vi "ImagingAndControl.vi"() -> ()   [LabVIEW 2015]
uses:
  <userlib>/atmcd64d.llb/Error Code Enum typedef.ctl
  <userlib>/atmcd64d.llb/HSSpeed_type typedef.ctl
  <vilib>/Analysis/baseanly.llb/Mean (DBL).vi
  AcquisitionGlobals.vi
  NIDAQControls/StateGlobals.vi
  NIDAQControls/NIDAQGlobals.vi
  LiveImage_Global.vi
  StartupVI_Globals.vi
  <userlib>/AB_ALC_REV64/AB_ALC_REV64.lvlib
  <vilib>/Analysis/NI_AALBase.lvlib
panel:
  out "gain":u32
  in  "Set EM Gain":u16(slide)=2995 min=3 max=300 scale=0.8..300.0
  in  "Live Volume":bool
  in  "max ypixels":i32=512
  in  "max xpixels":i32=512
  out "Saving?":bool
  out "Exposure Out":dbl=10.0
  out "start time":dbl format="%_19f"
  out "status":T1=enum."DRV_TEMPERATURE_STABILIZED"
  out "temperature":i32=-71
  in  "Acq Speed":u16(ring) items=["17", "10", "5", "1"]
  in  "Filter Position":i8=5
  out "Acquiring?":bool
  in  "ypixels":i32=512
  in  "xpixels":i32=512
  out "error out":errorcluster={"status"=FALSE, "code"=5002, "source"="ImagingAndControl.vi->GetAcquisitionTimings.vi"}
  in  "Tab Control":enum32{"Piezo Control", "Laser Control"}(tab)
  in  "Abort!":bool
  out "Recording time":dbl=16.0 format="%<%H:%M:%S%2u>t"
  out "Num Slices":u16=16
  in  "Waveform Type":enum16{"Triangle", "Sawtooth"}(ring)=enum."Sawtooth"
  in  "Center Piezo":bool
  out "Recording Progress":u8(slide) scale=0.0..100.0
  in  "Begin Acquisition":bool
  in  "File to Save":path=path "E:/maggot images/Jacob/Test/test_run143"
  in  "Acquisition Time (sec)":dbl=120.0
  in  "Volume On/Off":bool=TRUE
  out "Improper \nRange!":bool
  in  "Z Step Size (um)":dbl=0.8
  out "Current Z Position (um)":dbl=46.25
  in  "Max (um)":dbl=52.0
  in  "Min (um)":dbl=40.5
  in  "Set Min Piezo":bool
  in  "Set Max Piezo":bool
  out "Piezo Position":dbl(slide)=46.25 scale=0.0..100.0
  in  "Piezo Dwell":u16=1
  in  "Piezo Offset":dbl=-0.01
  out "Data Write Progress":u8(slide) scale=0.0..100.0
  in  "Trigger Mode":enum16{"Normal", "One Red Frame Per Volume"}(ring)=enum."One Red Frame Per Volume"
  in  "AOTF3 - 561 nm":dbl(slide)=21.02803738317757 scale=0.0..100.0
  in  "AOTF2 - 488 nm":dbl(slide)=20.560747663551403 scale=0.0..100.0
  in  "AOTF1 - 440 nm":dbl(slide) scale=0.0..100.0
  in  "Initialize Things?":bool
  out "Laser Mode":string="Confocal Green"
  in  "Live":bool
  in  "Exposure Time":T2(ring)
  in  "Triggered":bool
  in  "Confocal Red":bool
  in  "Confocal Green":bool=TRUE
  in  "Confocal Blue":bool
  out "LaserID":i32=2
  in  "stop":bool
  # ".h5"
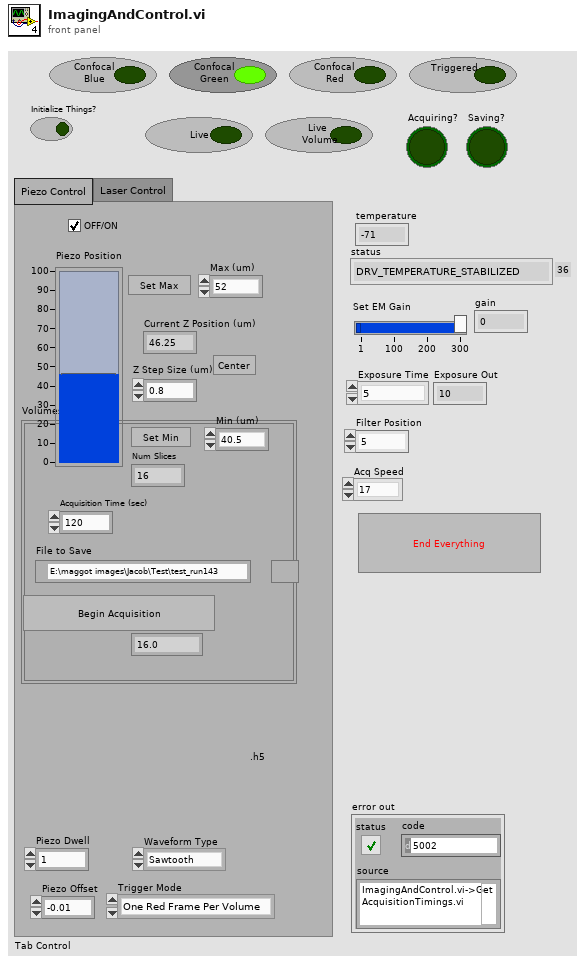
[diagram p1: front panel]
types:
  T1 = typedef "Error Code Enum typedef.ctl" = enum32{"N/A (0)", "DRV_ERROR_CODES", "DRV_SUCCESS", "DRV_VXDNOTINSTALLED", "DRV_ERROR_SCAN", "DRV_ERROR_CHECK_SUM", "DRV_ERROR_FILELOAD", "DRV_UNKNOWN_FUNC", "DRV_ERROR_VXD_INIT", "DRV_ERROR_ADDRESS", "DRV_ERROR_PAGELOCK", "DRV_ERROR_PAGEUNLOCK", "DRV_ERROR_BOARDTEST", "DRV_ERROR_ACK", "DRV_ERROR_UP_FIFO", "DRV_ERROR_PATTERN", "N/A (16)", "DRV_ACQUISITION_ERRORS", "DRV_ACQ_BUFFER", "DRV_ACQ_DOWNFIFO_FULL", "DRV_PROC_UNKONWN_INSTRUCTION", "DRV_ILLEGAL_OP_CODE", "DRV_KINETIC_TIME_NOT_MET", "DRV_ACCUM_TIME_NOT_MET", "DRV_NO_NEW_DATA", "N/A (25)", "DRV_SPOOLERROR", "N/A (27)", "N/A (28)", "N/A (29)", "N/A (30)", "N/A (31)", "N/A (32)", "DRV_TEMPERATURE_CODES", "DRV_TEMPERATURE_OFF", "DRV_TEMPERATURE_NOT_STABILIZED", "DRV_TEMPERATURE_STABILIZED", "DRV_TEMPERATURE_NOT_REACHED", "DRV_TEMPERATURE_OUT_RANGE", "DRV_TEMPERATURE_NOT_SUPPORTED", "DRV_TEMPERATURE_DRIFT", "N/A (41)", "N/A (42)", "N/A (43)", "N/A (44)", "N/A (45)", "N/A (46)", "N/A (47)", "N/A (48)", "DRV_GENERAL_ERRORS", "DRV_INVALID_AUX", "DRV_COF_NOTLOADED", "DRV_FPGAPROG", "DRV_FLEXERROR", "DRV_GPIBERROR", "N/A (55)", "N/A (56)", "N/A (57)", "N/A (58)", "N/A (59)", "N/A (60)", "N/A (61)", "N/A (62)", "N/A (63)", "DRV_DATATYPE", "DRV_DRIVER_ERRORS", "DRV_P1INVALID", "DRV_P2INVALID", "DRV_P3INVALID", "DRV_P4INVALID", "DRV_INIERROR", "DRV_COFERROR", "DRV_ACQUIRING", "DRV_IDLE", "DRV_TEMPCYCLE", "DRV_NOT_INITIALIZED", "DRV_P5INVALID", "DRV_P6INVALID", "DRV_INVALID_MODE", "DRV_INVALID_FILTER", "DRV_I2CERRORS", "DRV_I2CDEVNOTFOUND", "DRV_I2CTIMEOUT", "DRV_P7INVALID", "N/A (84)", "N/A (85)", "N/A (86)", "N/A (87)", "N/A (88)", "N/A (89)", "DRV_IOCERROR", "DRV_VRMVERSIONERROR"}
  T2 = enum16{"5", "10", "15", "20", "25", "30", "35", "40", "50", "60", "70", "100", "500"}
  T3 = cluster{"Start or New Parameters?":bool, "Laser Mode":string, "Piezo Mode":string, "Begin Or End Acquisition":string, "Acquisition Time":dbl}
  T4 = enum8{"Enabled", "Disabled", "Disabled and Grayed Out"}
  T5 = enum32{"Invalid", "Standard", "Closed", "Hidden", "Minimized", "Maximized"}
  T6 = typedef "HSSpeed_type typedef.ctl" = enum16{"EM Amp", "Conventional Amp"}
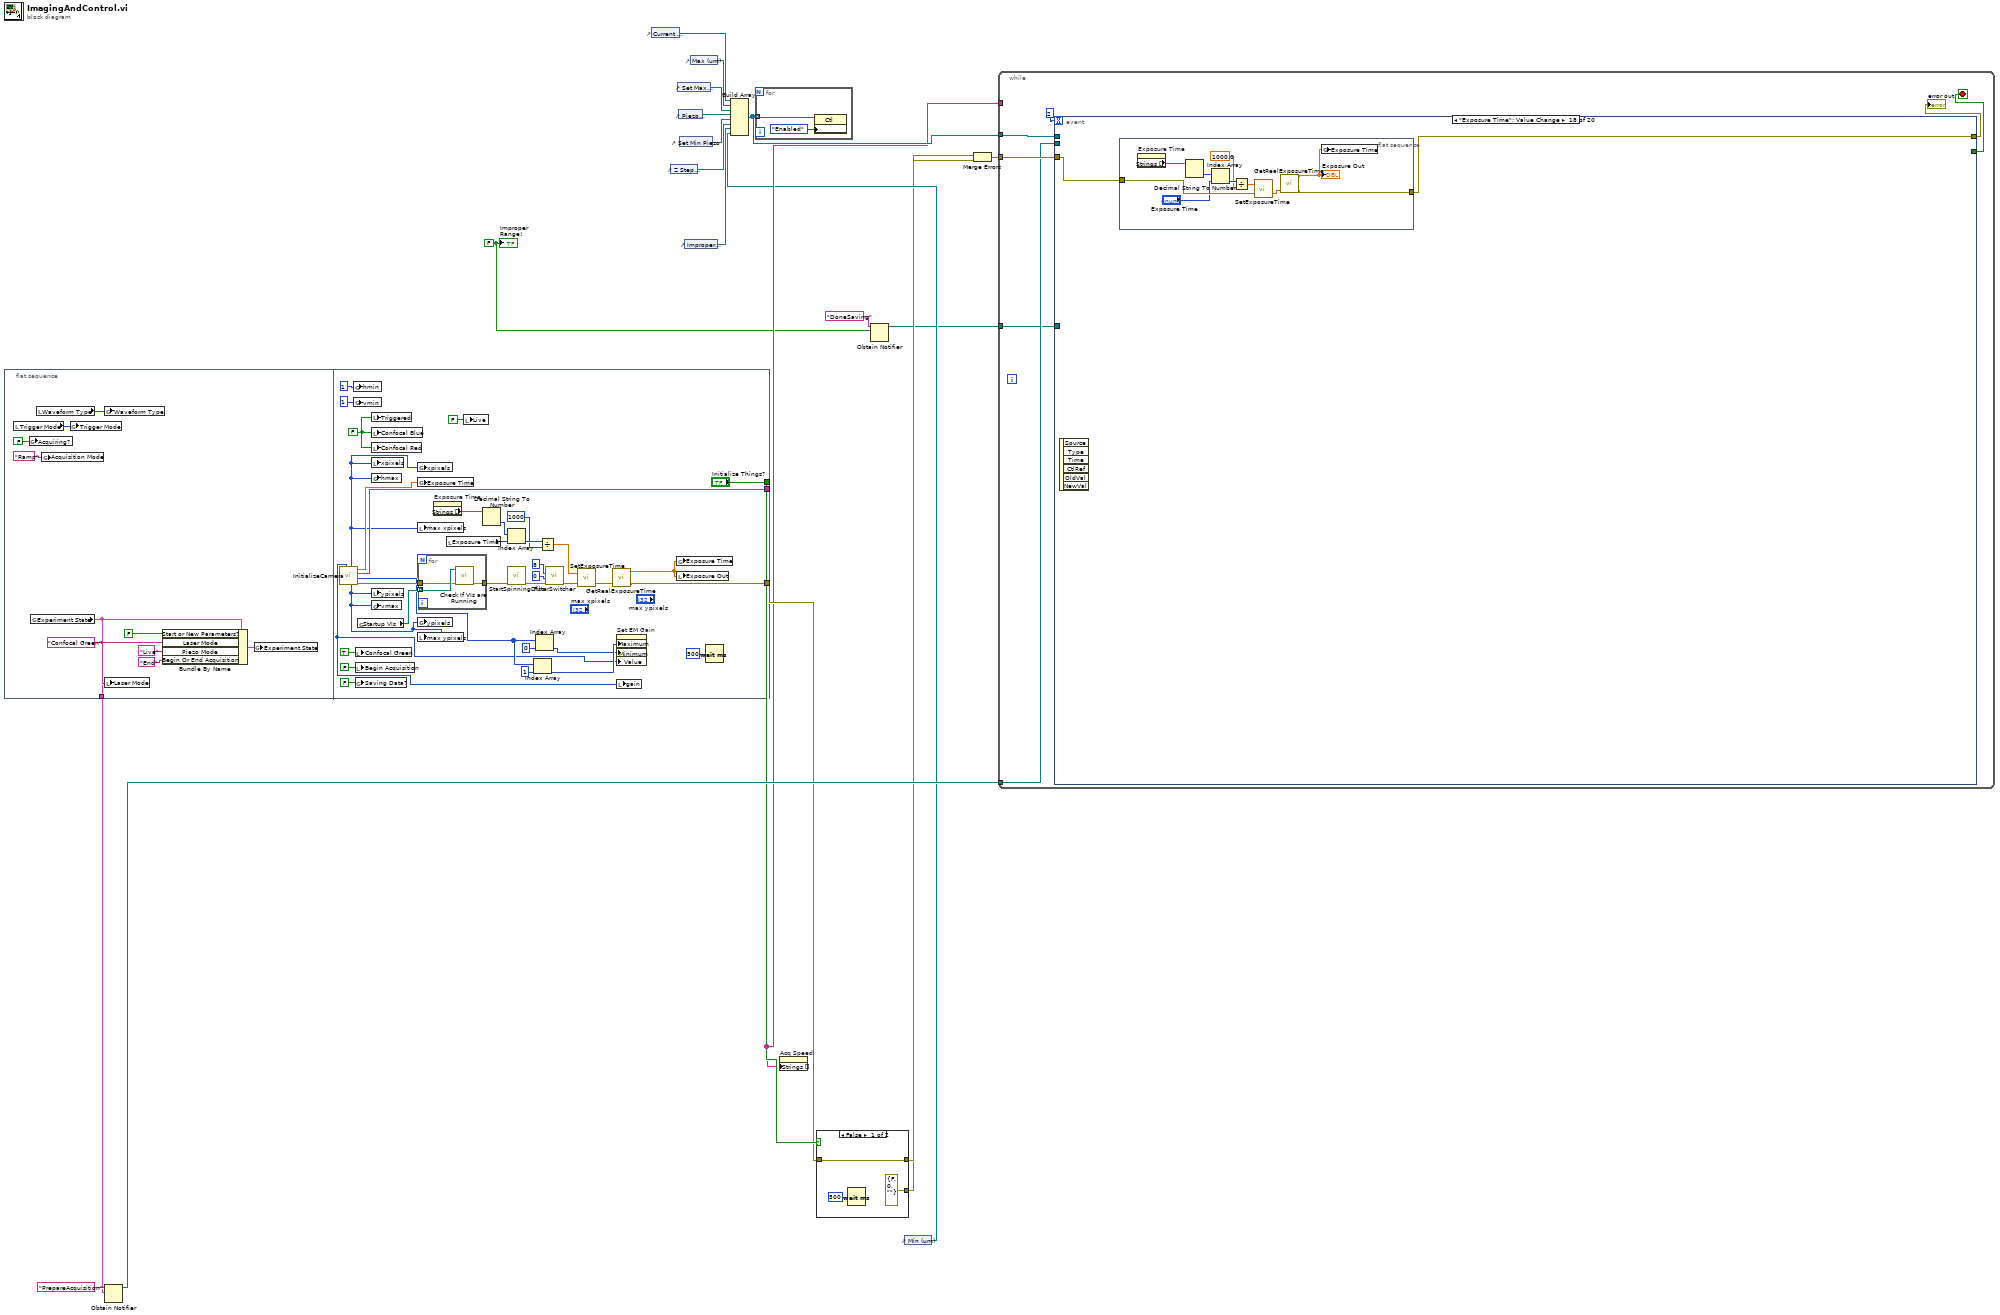
[diagram p0: block diagram]
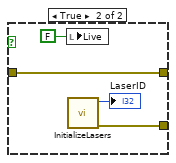
[diagram p2: hidden frame]
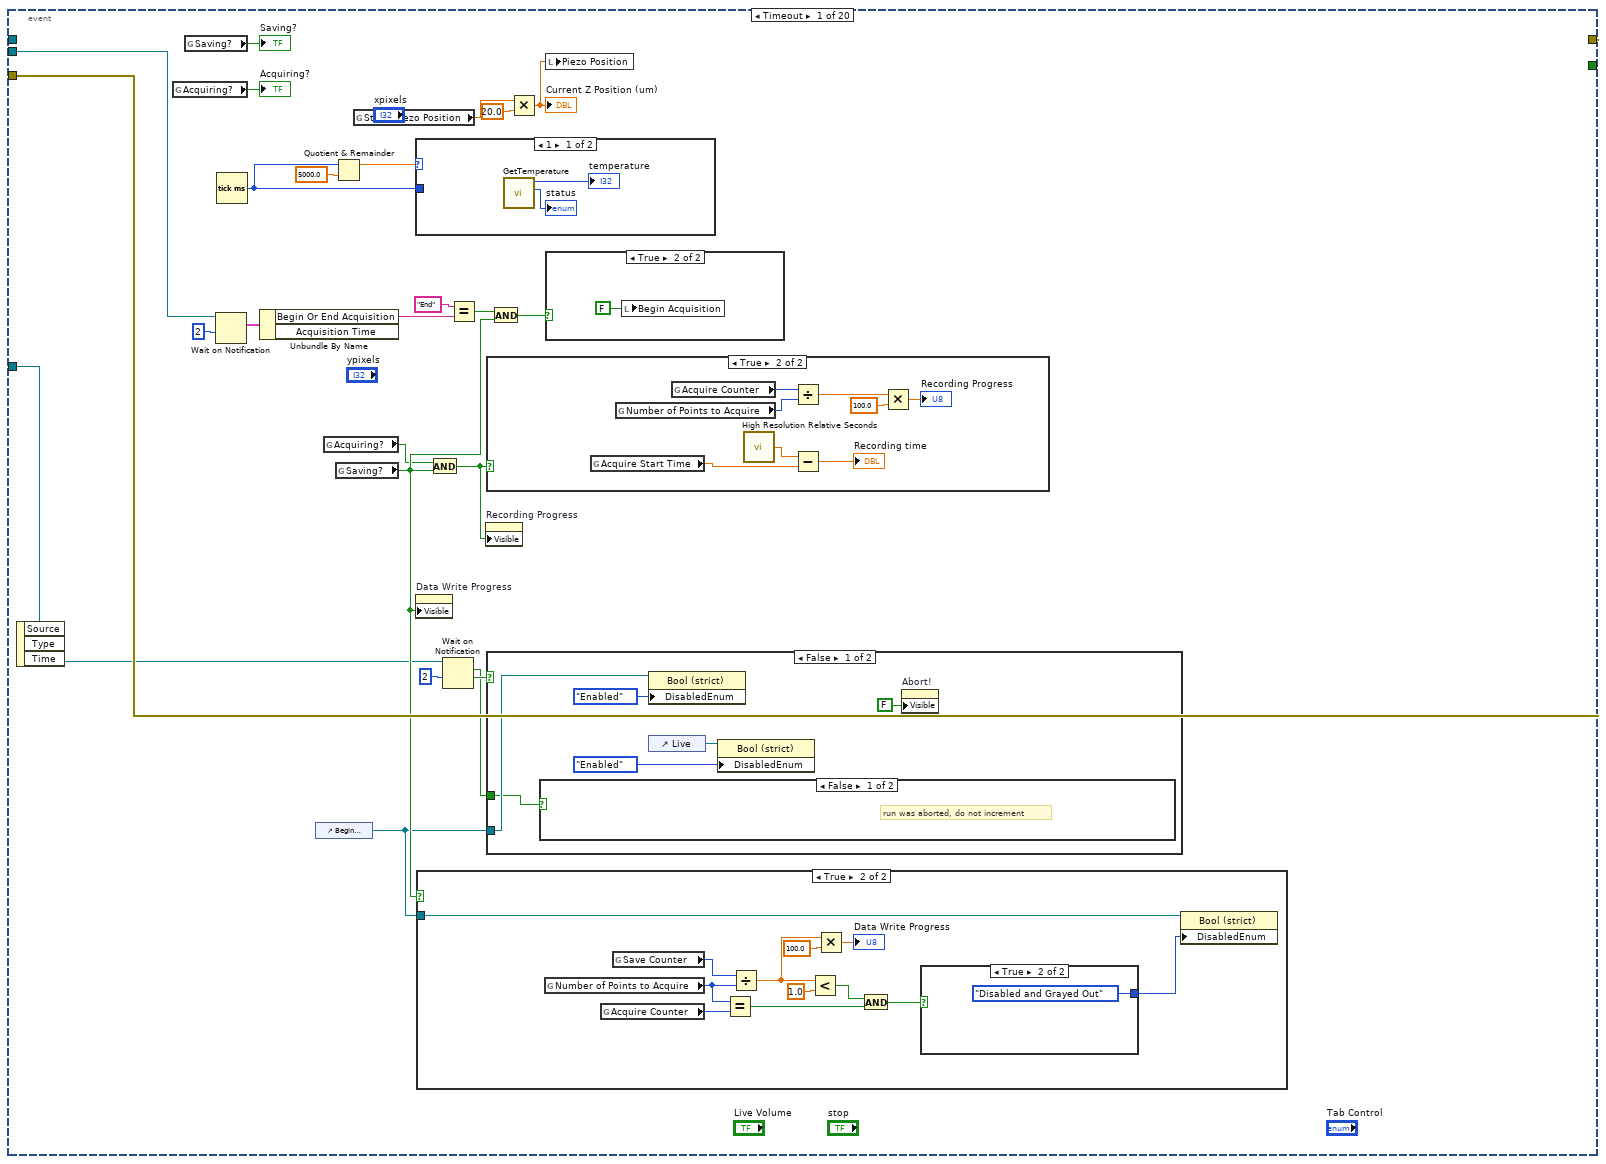
[diagram p3: hidden frame]
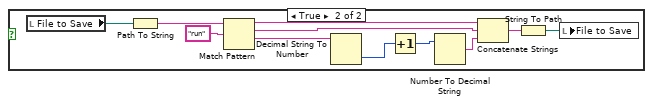
[diagram p4: hidden frame]
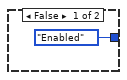
[diagram p8: hidden frame]
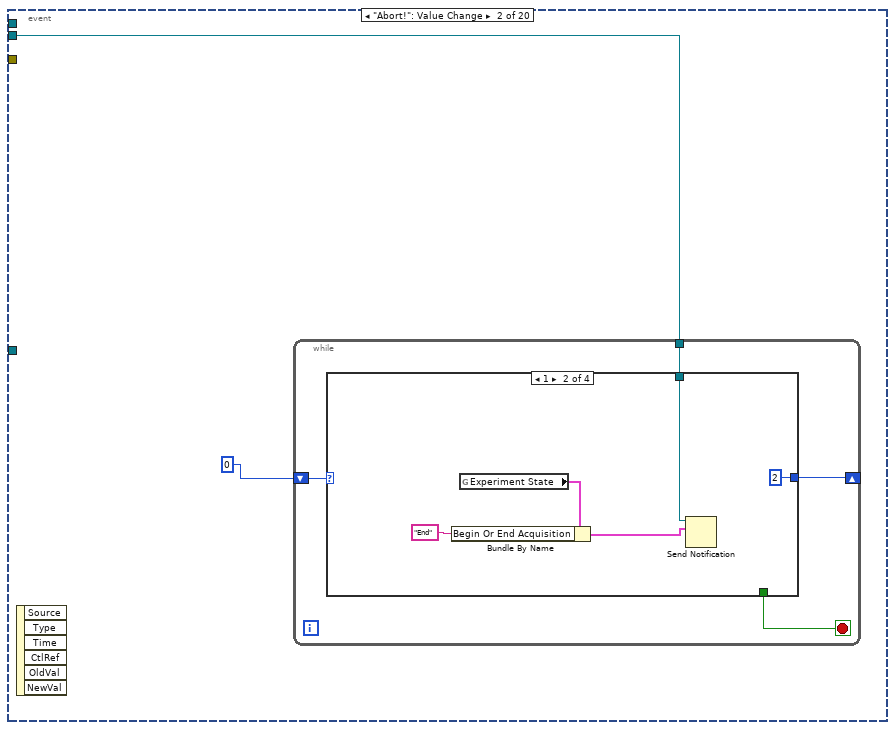
[diagram p11: hidden frame]
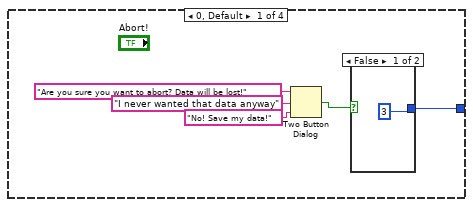
[diagram p12: hidden frame]
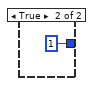
[diagram p13: hidden frame]
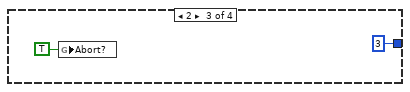
[diagram p14: hidden frame]
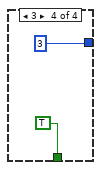
[diagram p15: hidden frame]
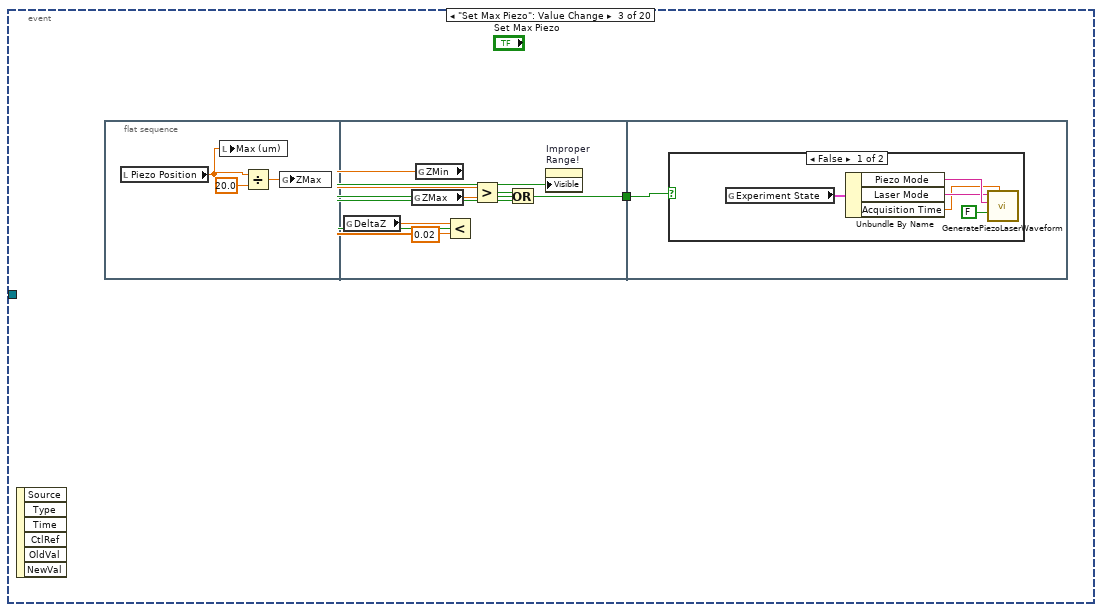
[diagram p16: hidden frame]
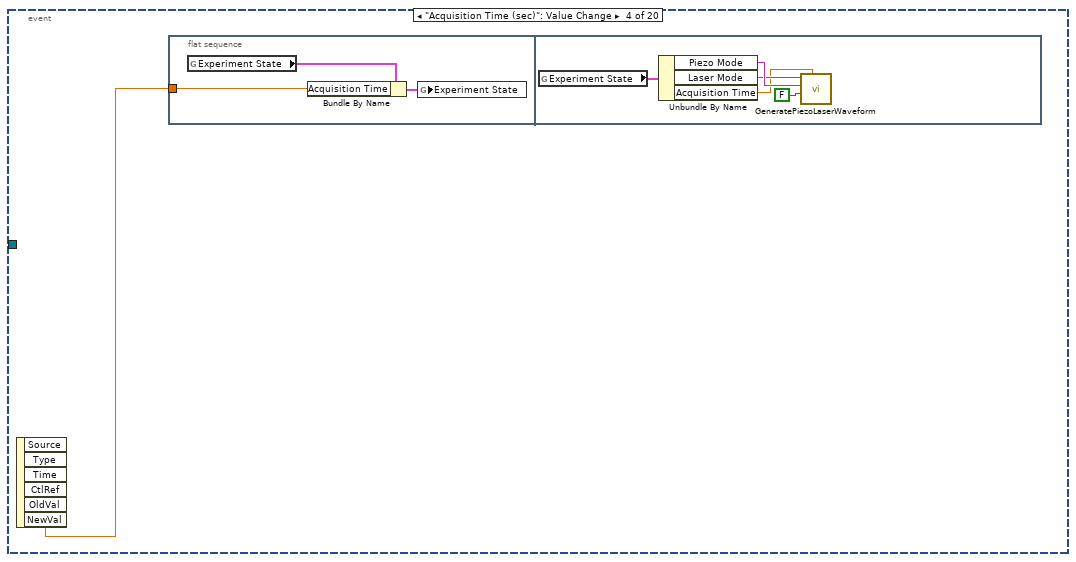
[diagram p18: hidden frame]
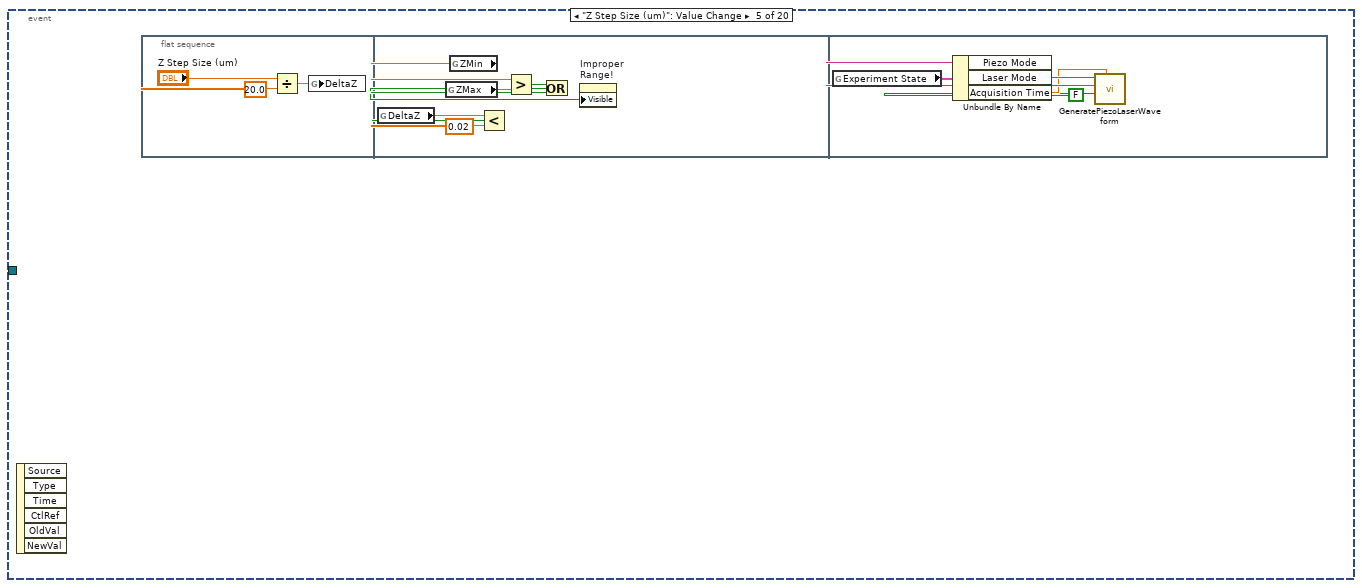
[diagram p19: hidden frame]
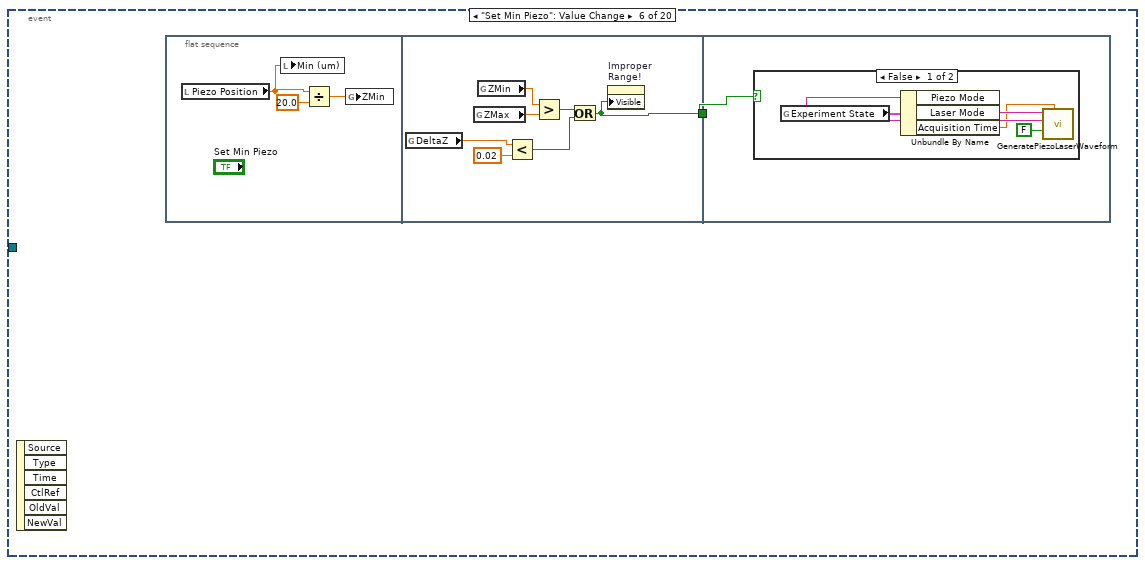
[diagram p20: hidden frame]
diagram:
  w2 = FALSE ("Improper \nRange!")
  n1 = flat-sequence {
    tunnel: [w24] -> w8
    tunnel: ["Initialize Things?"] -> w19
    tunnel: [w33] -> w10
    tunnel: [w56] -> w9
    frame #0 {
      w26 = "Confocal Green" ("Laser Mode")
      n2 = local read "Trigger Mode"() -> (w23:enum16{"Normal", "One Red Frame Per Volume"})
      n3 = global write "AcquisitionGlobals.vi" "Acquiring?"(FALSE ("Acquiring?")) -> ()
      n4 = global read "StateGlobals.vi" "Experiment State"() -> (w24:T3)
      n5 = local read "Waveform Type"() -> (w22:enum16{"Triangle", "Sawtooth"})
      n6 = global write "AcquisitionGlobals.vi" "Acquisition Mode"("Ramp" ("Acquisition Mode")) -> ()
      n7 = global write "NIDAQGlobals.vi" "Trigger Mode"(w23) -> ()
      n8 = global write "NIDAQGlobals.vi" "Waveform Type"(w22) -> ()
      n9 = local write "Laser Mode"(w26) -> ()
      n10 = Bundle By Name(cluster=w24, "Start or New Parameters?"=FALSE, "Laser Mode"=w26, "Piezo Mode"="Live", "Begin Or End Acquisition"="End") -> (w28:T3)
      n11 = global write "StateGlobals.vi" "Experiment State"(w28) -> ()
    }
    frame #1 {
      w61 = FALSE ("Confocal Blue")
      n12 = call "InitializeCamera.vi"() -> ("error out"=w64:errorcluster, "EM Gain Range"=w38:i32[], "EM Speeds"=w56:string[], "exposure time"=w60:sgl, "ypixels"=w52:i32, "xpixels"=w54:i32, "EM Gain"=w35:u32)  [unwired: 5 in]
      n13 = global write "LiveImage_Global.vi" "hmin"(1 ("hmin")) -> ()
      n14 = global write "LiveImage_Global.vi" "vmin"(1 ("vmin")) -> ()
      n15 = local write "Confocal Green"(TRUE ("Confocal Green")) -> ()
      n16 = local write "Begin Acquisition"(FALSE ("Begin Acquisition")) -> ()
      n17 = global write "AcquisitionGlobals.vi" "Saving Data?"(FALSE ("Saving Data?")) -> ()
      n18 = global read "StartupVI_Globals.vi" "Startup VIs"() -> (w65:path[])
      n19 = local write "Triggered"(w61) -> ()
      n20 = local write "Confocal Blue"(w61) -> ()
      n21 = local write "Confocal Red"(w61) -> ()
      n22 = local write "xpixels"(w54) -> ()
      n23 = global write "LiveImage_Global.vi" "hmax"(w54) -> ()
      n24 = local write "ypixels"(w52) -> ()
      n25 = global write "LiveImage_Global.vi" "vmax"(w52) -> ()
      n26 = global write "LiveImage_Global.vi" "xpixels"(w54) -> ()
      n27 = global write "LiveImage_Global.vi" "Exposure Time"(w60) -> ()
      n28 = local write "max xpixels"(w54) -> ()
      n29 = for {
        tunnel: w65 -> [w69] mode=indexing
        tunnel: w64 -> [w68]
        tunnel: [w67] -> w62
        n30 = call "Check If VIs are Running.vi"("error in (no error)"=w68, "Path"=w69) -> ("error out"=w67:errorcluster)  [unwired: 9 in]
      }
      n31 = global write "LiveImage_Global.vi" "ypixels"(w52) -> ()
      n32 = local write "max ypixels"(w52) -> ()
      n33 = property on="Exposure Time" class="Enum (strict)"() -> ("Strings []"=w47:string[])  [unwired: 2 in, 2 out]
      n34 = local read "Exposure Time"() -> (w46:T2)
      n35 = local write "Live"(FALSE ("Live")) -> ()
      n36 = Decimal String To Number(string=w47) -> (number=w49:i32[])  [unwired: 2 in, 1 out]
      n37 = Index Array(array=w49, index=w46) -> (element=w48:i32)
      n38 = call "StartSpinningDisc.vi"("error in (no error)"=w62) -> ("error out"=w59:errorcluster)  [unwired: 10 in]
      n39 = Index Array(array=w38, index=1) -> (element=w37:i32)
      n40 = Index Array(array=w38, index=0) -> (element=w36:i32)
      n41 = Divide(x=w48, y=1000) -> (x/y=w45:dbl)
      n42 = call "FilterSwitcher.vi"("error in (no error)"=w59, "Filter Change Speed"=0, "Filter Position"=8) -> ("error out"=w50:errorcluster)  [unwired: 8 in]
      n43 = call <userlib>:"SetExposureTime.vi"("error in (no error)"=w50, "time"=w45) -> ("error out"=w34:errorcluster)  [unwired: 1 out]
      n44 = call "GetRealExposureTime.vi"("error in (no error)"=w34) -> ("error out"=w33:errorcluster, "Actual Exposure Time (ms)"=w32:dbl)  [unwired: 9 in]
      n45 = property on="Set EM Gain" class="Slide (strict)"("Maximum"=w37, "Minimum"=w36, "Value"=w35) -> ()  [unwired: 2 in, 2 out]
      n46 = local write "gain"(w35) -> ()
      n47 = global write "LiveImage_Global.vi" "Exposure Time"(w32) -> ()
      n48 = local write "Exposure Out"(w32) -> ()
      n49 = Wait (ms)(milliseconds to wait=u32 500) -> ()  [unwired: 1 out]
    }
  }
  n50 = Obtain Notifier(name (unnamed)="PrepareAcquisition", notification data type=w8) -> (notifier out=w20:refnum<notifier>)  [unwired: 2 in, 2 out]
  n51 = control-ref of="Current Z Position (um)"() -> (w18:refnum<vi>)
  n52 = control-ref of="Z Step Size (um)"() -> (w13:refnum<vi>)
  n53 = control-ref of="Set Max Piezo"() -> (w16:refnum<vi>)
  n54 = control-ref of="Piezo Position"() -> (w15:refnum<vi>)
  n55 = control-ref of="Set Min Piezo"() -> (w14:refnum<vi>)
  n56 = control-ref of="Improper \nRange!"() -> (w12:refnum<vi>)
  n57 = control-ref of="Max (um)"() -> (w17:refnum<vi>)
  n58 = property on="Acq Speed" class="Ring (strict)"("Strings []"=w9) -> ()  [unwired: 2 in, 2 out]
  n59 = case shown="False" w19 {
    tunnel: [w71 w76] -> w6
    tunnel: [errorcluster {"status"=FALSE, "code"=0, "source"=""} ("error out") w75] -> w5
    tunnel: w10 -> [w71 w76]
    frame False {
      n60 = Wait (ms)(milliseconds to wait=u32 500) -> ()  [unwired: 1 out]
    }
    frame True {
      n61 = local write "Live"(FALSE ("Live")) -> ()
      n62 = call "InitializeLasers.vi"() -> ("error out"=w75:errorcluster, "hALC_REV out"=→"LaserID":i32)  [unwired: 10 in]
    }
  }
  n63 = Obtain Notifier(name (unnamed)="DoneSaving", notification data type=w2) -> (notifier out=w1:refnum<notifier>)  [unwired: 2 in, 2 out]
  n64 = control-ref of="Min (um)"() -> (w7:refnum<vi>)
  n65 = Build Array(w18, w17, w16, w15, w14, w13, w12, w7) -> (w11:refnum<vi>[])
  n66 = for {
    tunnel: w11 -> [w78] mode=indexing
    n67 = property class="Ctl"(reference=w78, "DisabledEnum"=T4."Enabled" ("Disabled")) -> ()  [unwired: 1 in, 2 out]
  }
  n68 = Merge Errors(w5, w6) -> (w4:errorcluster)
  n69 = while {
    tunnel: w4 -> [w85]
    tunnel: w20 -> [w84]
    tunnel: w11 -> [w82]
    tunnel: w9 -> [_]
    tunnel: w1 -> [w79]
    stop <- w81 stop-if-true
    n70 = event shown="[17] \"Exposure Time\": Value Change" {
      selector: _ -> [_ _ _ _ _ _ _ _ _ _ _ _ _ _ _ _ _ _ _ _]
      dyn-events: _ -> [_ _ _ _ _ _ _ _ _ _ _ _ _ _ _ _ _ _ _ _]
      timeout: 2 -> [_ _ _ _ _ _ _ _ _ _ _ _ _ _ _ _ _ _ _ _]
      tunnel: w85 -> [w94 _ _ _ _ _ w233 w263 w282 _ w308 w323 w326 w375 _ w442 _ w468 w483 _]
      tunnel: [w94 _ _ _ _ _ w232 w262 w281 _ w306 _ w324 w371 _ w441 _ w467 w483 _] -> w83
      tunnel: [_ _ _ _ _ _ _ _ _ _ w303 _ _ _ _ _ _ _ _ _] -> w81
      tunnel: w84 -> [w102 w152 _ _ _ _ w234 w264 w283 _ _ _ w325 w377 _ _ w449 _ w481 w503]
      tunnel: w82 -> [_ _ _ _ _ _ _ _ _ w296 _ _ _ _ _ _ _ _ _ _]
      tunnel: w79 -> [w90 _ _ _ _ _ _ _ _ _ _ _ _ _ _ _ _ _ _ _]
      event Timeout {
        n71 = event-data() -> ()  [unwired: 1 in, 3 out]
        n72 = global read "AcquisitionGlobals.vi" "Acquiring?"() -> (→"Acquiring?":bool)
        n73 = global read "AcquisitionGlobals.vi" "Saving?"() -> (→"Saving?":bool)
        n74 = Wait on Notification(notifier=w102, timeout in ms (-1)=2) -> (notification=w101:T3)  [unwired: 2 in, 3 out]
        n75 = Tick Count (ms)() -> (millisecond timer value=w105:u32)
        n76 = Unbundle By Name(w101) -> ("Begin Or End Acquisition"=w99:string)  [unwired: 1 out]
        n77 = control-ref of="Begin Acquisition"() -> (w87:refnum<vi>)
        n78 = global read "AcquisitionGlobals.vi" "Acquiring?"() -> (w92:bool)
        n79 = Quotient & Remainder(x=w105, y=5000.0) -> (x-y*floor(x/y)=w104:dbl)  [unwired: 1 out]
        n80 = global read "AcquisitionGlobals.vi" "Saving?"() -> (w93:bool)
        n81 = global read "NIDAQGlobals.vi" "Static Piezo Position"() -> (w109:dbl)
        n82 = case shown="1" w104 {
          tunnel: w105 -> [_ _]
          frame 1 {
            n83 = call <userlib>:"GetTemperature.vi"() -> ("status"=→"status":T1, "temperature"=→"temperature":i32)  [unwired: 4 in, 2 out]
          }
          frame 0, Default {
          }
        }
        n84 = property on="Data Write Progress" class="Slide (strict)"("Visible"=w93) -> ()  [unwired: 2 in, 2 out]
        n85 = case shown="True" w93 {
          tunnel: w87 -> [_ w135]
          frame False {
          }
          frame True {
            n86 = global read "StateGlobals.vi" "Number of Points to Acquire"() -> (w137:i32)
            n87 = global read "StateGlobals.vi" "Acquire Counter"() -> (w138:i32)
            n88 = global read "StateGlobals.vi" "Save Counter"() -> (w144:i32)
            n89 = Equal?(x=w137, y=w138) -> (x = y?=w140:bool)
            n90 = Divide(x=w144, y=w137) -> (x/y=w143:dbl)
            n91 = Less?(x=w143, y=1.0) -> (x < y?=w141:bool)
            n92 = Multiply(x=w143, y=100.0) -> (x*y=→"Data Write Progress":dbl)
            n93 = And(x=w141, y=w140) -> (x .and. y?=w139:bool)
            n94 = case shown="True" w139 {
              tunnel: [T4."Enabled" ("Disabled") T4."Disabled and Grayed Out" ("Disabled")] -> w136
              frame False {
              }
              frame True {
              }
            }
            n95 = property class="Bool (strict)"(reference=w135, "DisabledEnum"=w136) -> ()  [unwired: 1 in, 2 out]
          }
        }
        n96 = And(x=w92, y=w93) -> (x .and. y?=w91:bool)
        n97 = Wait on Notification(notifier=w90, timeout in ms (-1)=2) -> (notification=w86:bool, timed out?=w88:bool)  [unwired: 2 in, 2 out]
        n98 = Equal?(x="End", y=w99) -> (x = y?=w98:bool)
        n99 = property on="Recording Progress" class="Slide (strict)"("Visible"=w91) -> ()  [unwired: 2 in, 2 out]
        n100 = case shown="True" w91 {
          frame False {
          }
          frame True {
            n101 = global read "StateGlobals.vi" "Acquire Start Time"() -> (w129:dbl)
            n102 = global read "StateGlobals.vi" "Number of Points to Acquire"() -> (w128:i32)
            n103 = global read "StateGlobals.vi" "Acquire Counter"() -> (w127:i32)
            n104 = call <vilib>:"High Resolution Relative Seconds.vi"() -> ("relative seconds"=w134:dbl)
            n105 = Divide(x=w127, y=w128) -> (x/y=w130:dbl)
            n106 = Subtract(x=w134, y=w129) -> (x-y=→"Recording time":dbl)
            n107 = Multiply(x=w130, y=100.0) -> (x*y=→"Recording Progress":dbl)
          }
        }
        n108 = case shown="False" w88 {
          tunnel: w87 -> [w112 _]
          tunnel: w86 -> [w110 _]
          frame False {
            n109 = case shown="False" w110 {
              frame False {
                # "run was aborted, do not increment"
              }
              frame True {
                n110 = local read "File to Save"() -> (w116:path)
                n111 = Path To String(path=w116) -> (string=w118:string)
                n112 = Match Pattern(string=w118, regular expression="run") -> (before substring=w122:string, match substring=w123:string, after substring=w119:string)  [unwired: 1 in, 1 out]
                n113 = Decimal String To Number(string=w119) -> (number=w120:i32)  [unwired: 2 in, 1 out]
                n114 = Increment(x=w120) -> (x+1=w121:i32)
                n115 = Number To Decimal String(number=w121) -> (decimal integer string=w124:string)  [unwired: 1 in]
                n116 = Concatenate Strings(w122, w123, w124) -> (w125:string)
                n117 = String To Path(string=w125) -> (path=w126:path)
                n118 = local write "File to Save"(w126) -> ()
              }
            }
            n119 = property class="Bool (strict)"(reference=w112, "DisabledEnum"=T4."Enabled" ("Disabled")) -> ()  [unwired: 1 in, 2 out]
            n120 = control-ref of="Live"() -> (w113:refnum<vi>)
            n121 = property class="Bool (strict)"(reference=w113, "DisabledEnum"=T4."Enabled" ("Disabled")) -> ()  [unwired: 1 in, 2 out]
            n122 = property on="Abort!" class="Bool (strict)"("Visible"=FALSE) -> ()  [unwired: 2 in, 2 out]
          }
          frame True {
          }
        }
        n123 = And(x=w98, y=w93) -> (x .and. y?=w95:bool)
        n124 = Multiply(x=w109, y=20.0) -> (x*y=w107:dbl)
        "Current Z Position (um)" <- w107
        n125 = local write "Piezo Position"(w107) -> ()
        n126 = case shown="True" w95 {
          frame False {
          }
          frame True {
            n127 = local write "Begin Acquisition"(FALSE ("Begin Acquisition")) -> ()
          }
        }
      }
      event "Abort!": Value Change {
        n128 = event-data() -> ()  [unwired: 1 in, 6 out]
        n129 = while {
          shift-right: [w156] -> _
          shift-left: 0 -> [w157]
          tunnel: w152 -> [w154]
          stop <- w155 stop-if-true
          n130 = case shown="1" w157 {
            tunnel: [w158 2 3 3] -> w156
            tunnel: [_ _ _ TRUE] -> w155
            tunnel: w154 -> [_ w166 _ _]
            frame 0, Default {
              n131 = Two Button Dialog(message="Are you sure you want to abort? Data will be lost!", 1:"No! Save my data!" ("F button name (\"Cancel\")"), 2:"I never wanted that data anyway" ("T button name (\"OK\")")) -> (T button?=w159:bool)
              n132 = case shown="False" w159 {
                tunnel: [3 1] -> w158
                frame False {
                }
                frame True {
                }
              }
            }
            frame 1 {
              n133 = global read "StateGlobals.vi" "Experiment State"() -> (w167:T3)
              n134 = Bundle By Name(cluster=w167, "Begin Or End Acquisition"="End") -> (w169:T3)
              n135 = Send Notification(notification=w169, notifier=w166) -> ()  [unwired: 1 in, 2 out]
            }
            frame 2 {
              n136 = global write "AcquisitionGlobals.vi" "Abort?"(TRUE ("Abort?")) -> ()
            }
            frame 3 {
            }
          }
        }
      }
      event "Set Max Piezo": Value Change {
        n137 = event-data() -> ()  [unwired: 1 in, 6 out]
        n138 = flat-sequence {
          tunnel: [w178] -> w174
          tunnel: w174 -> [w185]
          frame #0 {
            n139 = local read "Piezo Position"() -> (w175:dbl)
            n140 = local write "Max (um)"(w175) -> ()
            n141 = Divide(x=w175, y=20.0) -> (x/y=w176:dbl)
            n142 = global write "NIDAQGlobals.vi" "ZMax"(w176) -> ()
          }
          frame #1 {
            n143 = global read "NIDAQGlobals.vi" "DeltaZ"() -> (w181:dbl)
            n144 = global read "NIDAQGlobals.vi" "ZMax"() -> (w183:dbl)
            n145 = global read "NIDAQGlobals.vi" "ZMin"() -> (w184:dbl)
            n146 = Less?(x=w181, y=0.02) -> (x < y?=w179:bool)
            n147 = Greater?(x=w184, y=w183) -> (0:w182:bool)
            n148 = Or(x=w182, y=w179) -> (x .or. y?=w178:bool)
            n149 = property on="Improper \nRange!" class="Bool (strict)"("Visible"=w178) -> ()  [unwired: 2 in, 2 out]
          }
          frame #2 {
            n150 = case shown="False" w185 {
              frame False {
                n151 = global read "StateGlobals.vi" "Experiment State"() -> (w190:T3)
                n152 = Unbundle By Name(w190) -> ("Piezo Mode"=w189:string, "Laser Mode"=w188:string, "Acquisition Time"=w187:dbl)
                n153 = call "GeneratePiezoLaserWaveform.vi"("Acquition Time (sec)"=w187, "Start or Continue?"=FALSE, "Piezo Mode"=w189, "Laser Mode"=w188) -> ()  [unwired: 5 in, 3 out]
              }
              frame True {
              }
            }
          }
        }
      }
      event "Acquisition Time (sec)": Value Change {
        n154 = event-data() -> ("NewVal"=w191:dbl)  [unwired: 1 in, 5 out]
        n155 = flat-sequence {
          tunnel: w191 -> [w193]
          frame #0 {
            n156 = global read "StateGlobals.vi" "Experiment State"() -> (w194:T3)
            n157 = Bundle By Name(cluster=w194, "Acquisition Time"=w193) -> (w192:T3)
            n158 = global write "StateGlobals.vi" "Experiment State"(w192) -> ()
          }
          frame #1 {
            n159 = global read "StateGlobals.vi" "Experiment State"() -> (w199:T3)
            n160 = Unbundle By Name(w199) -> ("Piezo Mode"=w198:string, "Laser Mode"=w197:string, "Acquisition Time"=w196:dbl)
            n161 = call "GeneratePiezoLaserWaveform.vi"("Acquition Time (sec)"=w196, "Start or Continue?"=FALSE, "Piezo Mode"=w198, "Laser Mode"=w197) -> ()  [unwired: 5 in, 3 out]
          }
        }
      }
      event "Z Step Size (um)": Value Change {
        n162 = event-data() -> ()  [unwired: 1 in, 6 out]
        n163 = flat-sequence {
          frame #0 {
            n164 = Divide(x="Z Step Size (um)", y=20.0) -> (x/y=w200:dbl)
            n165 = global write "NIDAQGlobals.vi" "DeltaZ"(w200) -> ()
          }
          frame #1 {
            n166 = global read "NIDAQGlobals.vi" "DeltaZ"() -> (w206:dbl)
            n167 = global read "NIDAQGlobals.vi" "ZMax"() -> (w208:dbl)
            n168 = global read "NIDAQGlobals.vi" "ZMin"() -> (w209:dbl)
            n169 = Less?(x=w206, y=0.02) -> (x < y?=w204:bool)
            n170 = Greater?(x=w209, y=w208) -> (0:w207:bool)
            n171 = Or(x=w207, y=w204) -> (x .or. y?=w203:bool)
            n172 = property on="Improper \nRange!" class="Bool (strict)"("Visible"=w203) -> ()  [unwired: 2 in, 2 out]
          }
          frame #2 {
            n173 = global read "StateGlobals.vi" "Experiment State"() -> (w214:T3)
            n174 = Unbundle By Name(w214) -> ("Piezo Mode"=w213:string, "Laser Mode"=w212:string, "Acquisition Time"=w211:dbl)
            n175 = call "GeneratePiezoLaserWaveform.vi"("Acquition Time (sec)"=w211, "Start or Continue?"=FALSE, "Piezo Mode"=w213, "Laser Mode"=w212) -> ()  [unwired: 5 in, 3 out]
          }
        }
      }
      event "Set Min Piezo": Value Change {
        n176 = event-data() -> ()  [unwired: 1 in, 6 out]
        n177 = flat-sequence {
          tunnel: [w219] -> w215
          tunnel: w215 -> [w226]
          frame #0 {
            n178 = local read "Piezo Position"() -> (w216:dbl)
            n179 = local write "Min (um)"(w216) -> ()
            n180 = Divide(x=w216, y=20.0) -> (x/y=w217:dbl)
            n181 = global write "NIDAQGlobals.vi" "ZMin"(w217) -> ()
          }
          frame #1 {
            n182 = global read "NIDAQGlobals.vi" "DeltaZ"() -> (w222:dbl)
            n183 = global read "NIDAQGlobals.vi" "ZMax"() -> (w224:dbl)
            n184 = global read "NIDAQGlobals.vi" "ZMin"() -> (w225:dbl)
            n185 = Less?(x=w222, y=0.02) -> (x < y?=w220:bool)
            n186 = Greater?(x=w225, y=w224) -> (0:w223:bool)
            n187 = Or(x=w223, y=w220) -> (x .or. y?=w219:bool)
            n188 = property on="Improper \nRange!" class="Bool (strict)"("Visible"=w219) -> ()  [unwired: 2 in, 2 out]
          }
          frame #2 {
            n189 = case shown="False" w226 {
              frame False {
                n190 = global read "StateGlobals.vi" "Experiment State"() -> (w231:T3)
                n191 = Unbundle By Name(w231) -> ("Piezo Mode"=w230:string, "Laser Mode"=w229:string, "Acquisition Time"=w228:dbl)
                n192 = call "GeneratePiezoLaserWaveform.vi"("Acquition Time (sec)"=w228, "Start or Continue?"=FALSE, "Piezo Mode"=w230, "Laser Mode"=w229) -> ()  [unwired: 5 in, 3 out]
              }
              frame True {
              }
            }
          }
        }
      }
      event "Max (um)", "Min (um)", "Piezo Dwell", "Piezo Offset": Value Change {
        n193 = event-data() -> ()  [unwired: 1 in, 6 out]
        n194 = flat-sequence {
          tunnel: w234 -> [w256]
          tunnel: w233 -> [w255]
          tunnel: [w254] -> w232
          frame #0 {
            w242 = 20.0 ("y")
            n195 = Divide(x="Min (um)", y=w242) -> (x/y=w241:dbl)
            n196 = Divide(x="Max (um)", y=w242) -> (x/y=w236:dbl)
            n197 = global write "NIDAQGlobals.vi" "ZMin"(w241) -> ()
            n198 = global write "NIDAQGlobals.vi" "ZMax"(w236) -> ()
            n199 = global read "NIDAQGlobals.vi" "DeltaZ"() -> (w246:dbl)
            n200 = control-ref of="Improper \nRange!"() -> (w240:refnum<vi>)
            n201 = Greater Or Equal?(x=w241, y=w236) -> (x >= y?=w247:bool)
            n202 = Less?(x=w246, y=0.02) -> (x < y?=w245:bool)
            n203 = Or(x=w247, y=w245) -> (x .or. y?=w244:bool)
            n204 = global write "NIDAQGlobals.vi" "Dwell"("Piezo Dwell") -> ()
            n205 = case shown="False" w244 {
              frame False {
                n206 = global read "StateGlobals.vi" "Experiment State"() -> (w252:T3)
                n207 = Unbundle By Name(w252) -> ("Laser Mode"=w251:string, "Acquisition Time"=w250:dbl)  [unwired: 1 out]
                n208 = call "GeneratePiezoLaserWaveform.vi"("Acquition Time (sec)"=w250, "Start or Continue?"=FALSE, "Piezo Mode"="Ramp", "Laser Mode"=w251) -> ()  [unwired: 5 in, 3 out]
              }
              frame True {
              }
            }
            n209 = property on="Property Node" class="Bool (strict)"(reference=w240, "Visible"=w244) -> ()  [unwired: 1 in, 2 out]
            n210 = global write "NIDAQGlobals.vi" "Offset"("Piezo Offset") -> ()
          }
          frame #1 {
            n211 = local read "Live Volume"() -> (w257:bool)
            n212 = case shown="True" w257 {
              tunnel: w256 -> [_ w259]
              tunnel: w255 -> [_ w260]
              tunnel: [_ w258] -> w254
              frame False {
              }
              frame True {
                n213 = call "RestartImagingWNewParameters.vi"("error IO"=w260, "notifier out"=w259) -> ("error out 2"=w258:errorcluster)  [unwired: 9 in]
              }
            }
            n214 = global read "NIDAQGlobals.vi" "Volume Size"() -> (→"Num Slices":u16)
          }
        }
      }
      event "Center Piezo": Value Change {
        n215 = event-data() -> ()  [unwired: 1 in, 6 out]
        n216 = flat-sequence {
          tunnel: w263 -> [w272]
          tunnel: [w272] -> w261
          tunnel: w264 -> [w275]
          tunnel: [w273] -> w262
          tunnel: w261 -> [w274]
          frame #0 {
            w267 = 20.0 ("y")
            n217 = global read "NIDAQGlobals.vi" "ZMax"() -> (w270:dbl)
            n218 = global read "NIDAQGlobals.vi" "ZMin"() -> (w271:dbl)
            n219 = Build Array(w271, w270) -> (w266:dbl[])
            n220 = Multiply(x=w266, y=w267) -> (x*y=w265:dbl[])
            n221 = call-poly <vilib>:"Mean.vi"("X"=w265) -> ("mean"=w269:dbl)  [unwired: 1 out]
            n222 = local write "Current Z Position (um)"(w269) -> ()
            n223 = local write "Piezo Position"(w269) -> ()
            n224 = Divide(x=w269, y=w267) -> (x/y=w268:dbl)
            n225 = global write "NIDAQGlobals.vi" "Static Piezo Position"(w268) -> ()
          }
          frame #1 {
            n226 = local read "Live Volume"() -> (w276:bool)
            n227 = case shown="True" w276 {
              tunnel: w275 -> [_ w278]
              tunnel: w274 -> [_ w279]
              tunnel: [_ w277] -> w273
              frame False {
              }
              frame True {
                n228 = call "RestartImagingWNewParameters.vi"("error IO"=w279, "notifier out"=w278) -> ("error out 2"=w277:errorcluster)  [unwired: 9 in]
              }
            }
          }
        }
      }
      event "Waveform Type", "Trigger Mode": Value Change {
        n229 = event-data() -> ()  [unwired: 1 in, 6 out]
        n230 = flat-sequence {
          tunnel: w282 -> [w286]
          tunnel: [w286] -> w280
          tunnel: w283 -> [w289]
          tunnel: [w287] -> w281
          tunnel: w280 -> [w288]
          frame #0 {
            n231 = global write "NIDAQGlobals.vi" "Waveform Type"("Waveform Type") -> ()
            n232 = global write "NIDAQGlobals.vi" "Trigger Mode"("Trigger Mode") -> ()
          }
          frame #1 {
            n233 = local read "Live Volume"() -> (w290:bool)
            n234 = case shown="True" w290 {
              tunnel: w289 -> [_ w292]
              tunnel: w288 -> [_ w293]
              tunnel: [_ w291] -> w287
              frame False {
              }
              frame True {
                n235 = call "RestartImagingWNewParameters.vi"("error IO"=w293, "notifier out"=w292) -> ("error out 2"=w291:errorcluster)  [unwired: 9 in]
              }
            }
          }
        }
      }
      event "Volume On/Off": Value Change {
        n236 = event-data() -> ()  [unwired: 1 in, 6 out]
        n237 = case shown="True" "Volume On/Off" {
          tunnel: [T4."Disabled and Grayed Out" ("Disabled") T4."Enabled" ("Disabled")] -> w294
          frame False {
            n238 = global write "AcquisitionGlobals.vi" "Acquisition Mode"("Live" ("Acquisition Mode")) -> ()
          }
          frame True {
            n239 = global write "AcquisitionGlobals.vi" "Acquisition Mode"("Ramp" ("Acquisition Mode")) -> ()
          }
        }
        n240 = for {
          tunnel: w296 -> [w302] mode=indexing
          tunnel: w294 -> [w301]
          n241 = property class="Ctl"(reference=w302, "DisabledEnum"=w301) -> ()  [unwired: 1 in, 2 out]
        }
      }
      event "stop": Value Change {
        n242 = event-data() -> ()  [unwired: 1 in, 6 out]
        n243 = local read "LaserID"() -> (w304:i32)
        n244 = flat-sequence {
          tunnel: w308 -> [w314]
          tunnel: [w313] -> w307
          tunnel: w304 -> [w311]
          tunnel: w307 -> [w317]
          tunnel: [w315] -> w305
          tunnel: [w319] -> w306
          tunnel: w305 -> [w319]
          tunnel: [TRUE] -> w303
          frame #0 {
            n245 = call <userlib>:"Delete ALC REV C.vi"("error in (no error)"=w314, "hALC_REV"=w311) -> ("error out"=w313:errorcluster, "function return"=w312:i32)  [unwired: 8 in]
            n246 = Equal?(x=w312, y=0) -> ()  [unwired: 1 out]
            n247 = Wait (ms)(milliseconds to wait=u32 500) -> ()  [unwired: 1 out]
          }
          frame #1 {
            n248 = call <userlib>:"CoolerOFF.vi"("error in (no error)"=w317) -> ("error out"=w316:errorcluster)  [unwired: 1 in, 1 out]
            n249 = call <userlib>:"ShutDown.vi"("error in (no error)"=w316) -> ("error out"=w315:errorcluster)  [unwired: 1 in, 1 out]
          }
          frame #2 {
          }
        }
      }
      event "Set EM Gain": Value Change {
        n250 = event-data() -> ()  [unwired: 1 in, 6 out]
        n251 = call <userlib>:"SetEMCCDGain.vi"("error in (no error)"=w323, "gain"="Set EM Gain") -> ("error out"=w321:errorcluster)  [unwired: 1 out]
        n252 = call <userlib>:"GetEMCCDGain.vi"("error in (no error)"=w321) -> ("gain"=→"gain":u32)  [unwired: 2 in, 2 out]
      }
      event "Confocal Blue", "Confocal Green", "Confocal Red", "Triggered": Value Change {
        n253 = event-data() -> ("CtlRef"=w327:refnum<vi>)  [unwired: 1 in, 5 out]
        n254 = flat-sequence {
          tunnel: w327 -> [w352]
          tunnel: w326 -> [w345]
          tunnel: w325 -> [w342]
          tunnel: [w339] -> w324
          frame #0 {
            n255 = property class="Bool (strict)"(reference=w352) -> ("Label.Text"=w343:string)  [unwired: 1 in, 2 out]
            "Laser Mode" <- w343
            n256 = global read "StateGlobals.vi" "Experiment State"() -> (w338:T3)
            n257 = case shown="\"Triggered\"" w343 {
              tunnel: TRUE -> [w358 w362 w365 w369]
              tunnel: [w358 w361 w366 w370] -> w351
              tunnel: [w357 w362 w366 w370] -> w350
              tunnel: [w357 w361 w365 w370] -> w349
              tunnel: [w357 w361 w366 w369] -> w348
              tunnel: FALSE -> [w357 w361 w366 w370]
              tunnel: [w356 w360 w364 w368] -> w344
              tunnel: [1 i8 1 0 5] -> w328
              frame "Confocal Blue" {
                w356 = u16 1 items=["1", "2", "3"] ("Ring")
              }
              frame "Confocal Green", Default {
                w360 = u16 0 items=["1", "2", "3"] ("Ring")
              }
              frame "Confocal Red" {
                w364 = u16 1 items=["1", "2", "3"] ("Ring")
              }
              frame "Triggered" {
                w368 = u16 1 items=["1", "2", "3"] ("Ring")
              }
            }
            n258 = Unbundle By Name(w338) -> ("Piezo Mode"=w337:string, "Begin Or End Acquisition"=w336:string)  [unwired: 2 out]
            n259 = Bundle By Name(cluster=w338, "Start or New Parameters?"=FALSE, "Laser Mode"=w343, "Piezo Mode"=w337, "Begin Or End Acquisition"=w336) -> (w329:T3)
            n260 = local write "Triggered"(w348) -> ()
            n261 = global write "StateGlobals.vi" "Experiment State"(w329) -> ()
            n262 = Unbundle By Name(w329) -> ("Piezo Mode"=w333:string, "Laser Mode"=w332:string, "Acquisition Time"=w331:dbl)
            n263 = local write "Confocal Red"(w349) -> ()
            n264 = local write "Confocal Green"(w350) -> ()
            n265 = local write "Confocal Blue"(w351) -> ()
            n266 = global read "AcquisitionGlobals.vi" "Acquiring?"() -> (w334:bool)
            n267 = call "CubeSwitcher.vi"("error in (no error)"=w345, "Ring"=w344) -> ("error out"=w341:errorcluster)  [unwired: 9 in]
            n268 = case shown="True" w334 {
              tunnel: w342 -> [_ w354]
              tunnel: w329 -> [_ w353]
              frame False {
              }
              frame True {
                n269 = Send Notification(notification=w353, notifier=w354) -> ()  [unwired: 1 in, 2 out]
              }
            }
            n270 = call "GeneratePiezoLaserWaveform.vi"("Acquition Time (sec)"=w331, "Start or Continue?"=FALSE, "Piezo Mode"=w333, "Laser Mode"=w332) -> ()  [unwired: 5 in, 3 out]
            n271 = call "FilterSwitcher.vi"("error in (no error)"=w341, "Filter Change Speed"=0, "Filter Position"=w328) -> ("error out"=w339:errorcluster)  [unwired: 8 in]
            n272 = local write "Filter Position"(w328) -> ()
          }
        }
      }
      event "Begin Acquisition", "Live", "Live Volume": Value Change {
        # "Live Volume Case"
        n273 = event-data() -> ("CtlRef"=w380:refnum<vi>, "NewVal"=w378:bool)  [unwired: 1 in, 4 out]
        n274 = flat-sequence {
          tunnel: w380 -> [w412]
          tunnel: w378 -> [w382]
          tunnel: [w408] -> w379
          tunnel: [w385] -> _
          tunnel: w375 -> [w390]
          tunnel: [w390] -> w376
          tunnel: w379 -> [w437]
          tunnel: [w438] -> w372
          tunnel: w377 -> [w436]
          tunnel: w376 -> [w435]
          frame #0 {
            w391 = T4."Enabled" ("Disabled")
            n275 = property class="Bool (strict)"(reference=w412) -> ("Label.Text"=w385:string)  [unwired: 1 in, 2 out]
            n276 = Path To String(path="File to Save") -> (string=w406:string)
            n277 = Concatenate Strings(w406, ".h5" ("string")) -> (w404:string)
            n278 = String To Path(string=w404) -> (path=w403:path)
            n279 = case shown="\"Begin Acquisition\"" w385 {
              tunnel: [w423 "Live" ("Piezo Mode") w432] -> w399
              tunnel: ["Acquisition Time (sec)" 0.0 ("Acquisition Time (0 for live)") 10.0 ("Acquisition Time (0 for live)")] -> w401
              tunnel: [TRUE ("Saving Data?") w425 FALSE ("Saving Data?")] -> w386
              tunnel: w391 -> [w420 w426 _]
              tunnel: [w419 w426 w431] -> w397
              tunnel: T4."Disabled and Grayed Out" ("Disabled") -> [w419 w427 w431]
              tunnel: [w420 w427 w431] -> w392
              tunnel: [TRUE ("Saving Data?") w425 TRUE ("Saving Data?")] -> w388
              frame "Begin Acquisition" {
                n280 = call <vilib>:"High Resolution Relative Seconds.vi"() -> ("relative seconds"=→"start time":dbl)
                n281 = global read "AcquisitionGlobals.vi" "Acquisition Mode"() -> (w423:string)
              }
              frame "Live", Default {
                w425 = FALSE ("Saving Data?")
              }
              frame "Live Volume" {
                n282 = global read "AcquisitionGlobals.vi" "Acquisition Mode"() -> (w432:string)
              }
            }
            n283 = global write "AcquisitionGlobals.vi" "File Save Path"(w403) -> ()
            n284 = Equal?(x=w385, y="Begin Acquisition") -> (x = y?=w383:bool)
            n285 = And(x=w382, y=w383) -> (x .and. y?=w381:bool)
            n286 = local read "Volume On/Off"() -> (w389:bool)
            n287 = local read "Laser Mode"() -> (w400:string)
            n288 = property on="Abort!" class="Bool (strict)"("Visible"=w381) -> ()  [unwired: 2 in, 2 out]
            n289 = case shown="False" w382 {
              tunnel: ["End" ("Begin Or End Acquisition") "Begin" ("Begin Or End Acquisition")] -> w410
              tunnel: w397 -> [_ w415]
              tunnel: [w413 w416] -> w394
              tunnel: [w413 w415] -> w395
              tunnel: w392 -> [_ w416]
              tunnel: w391 -> [w413 _]
              frame False {
              }
              frame True {
              }
            }
            n290 = global write "AcquisitionGlobals.vi" "Saving Data?"(w386) -> ()
            n291 = And(x=w389, y=w388) -> (x .and. y?=w387:bool)
            n292 = call "GeneratePiezoLaserWaveform.vi"("Acquition Time (sec)"=w401, "Start or Continue?"=FALSE, "Piezo Mode"=w399, "Laser Mode"=w400) -> ()  [unwired: 5 in, 3 out]
            n293 = global read "StateGlobals.vi" "Experiment State"() -> (w411:T3)
            n294 = global write "AcquisitionGlobals.vi" "Volumes?"(w387) -> ()
            n295 = control-ref of="Begin Acquisition"() -> (w398:refnum<vi>)
            n296 = property class="Bool (strict)"(reference=w398, "DisabledEnum"=w394) -> ()  [unwired: 1 in, 2 out]
            n297 = control-ref of="Live"() -> (w396:refnum<vi>)
            n298 = Bundle By Name(cluster=w411, "Start or New Parameters?"=TRUE, "Laser Mode"=w400, "Piezo Mode"=w399, "Begin Or End Acquisition"=w410, "Acquisition Time"=w401) -> (w408:T3)
            n299 = property class="Bool (strict)"(reference=w396, "DisabledEnum"=w395) -> ()  [unwired: 1 in, 2 out]
            n300 = global write "StateGlobals.vi" "Experiment State"(w408) -> ()
          }
          frame #1 {
            n301 = Send Notification(notification=w437, notifier=w436, error in (no error)=w435) -> (error out=w438:errorcluster)  [unwired: 1 out]
          }
        }
        n302 = call "Check If VIs are Running.vi"("error in (no error)"=w372, "State"=T5."Standard", "Path"=path "C:/Users/Public/Documents/National Instruments/AndorAcquire/Andor/LiveVolumeImaging.vi") -> ("error out"=w371:errorcluster)  [unwired: 8 in]
      }
      event "Filter Position": Value Change {
        n303 = event-data() -> ()  [unwired: 1 in, 6 out]
        n304 = flat-sequence {
          frame #0 {
            n305 = call "FilterSwitcher.vi"("Filter Change Speed"=0, "Filter Position"="Filter Position") -> ()  [unwired: 9 in, 1 out]
          }
        }
      }
      event "Acq Speed": Value Change {
        n306 = event-data() -> ()  [unwired: 1 in, 6 out]
        n307 = flat-sequence {
          tunnel: w442 -> [w444]
          tunnel: [w443] -> w441
          frame #0 {
            n308 = call <userlib>:"SetHSSpeed.vi"("error in (no error)"=w444, "index"="Acq Speed", "type"=HSSpeed_type_typedef."EM Amp") -> ("error out"=w443:errorcluster)  [unwired: 1 in, 1 out]
          }
        }
      }
      event "AOTF1 - 440 nm", "AOTF2 - 488 nm", "AOTF3 - 561 nm": Value Change {
        n309 = event-data() -> ()  [unwired: 1 in, 6 out]
        n310 = flat-sequence {
          tunnel: [w451] -> w448
          tunnel: [w450] -> w447
          tunnel: w449 -> [w464]
          tunnel: w448 -> [w463]
          tunnel: w447 -> [w462]
          frame #0 {
            w460 = 20.0 ("y")
            n311 = global read "StateGlobals.vi" "Experiment State"() -> (w453:T3)
            n312 = Divide(x="AOTF1 - 440 nm", y=w460) -> (x/y=w455:dbl)
            n313 = Divide(x="AOTF2 - 488 nm", y=w460) -> (x/y=w456:dbl)
            n314 = Divide(x="AOTF3 - 561 nm", y=w460) -> (x/y=w457:dbl)
            n315 = global write "NIDAQGlobals.vi" "Blue"(w455) -> ()
            n316 = Bundle By Name(cluster=w453, "Start or New Parameters?"=FALSE, "Begin Or End Acquisition"="ChangeDaq") -> (w451:T3)
            n317 = global write "NIDAQGlobals.vi" "Green"(w456) -> ()
            n318 = global write "NIDAQGlobals.vi" "Red"(w457) -> ()
            n319 = global write "StateGlobals.vi" "Experiment State"(w451) -> ()
            n320 = global read "AcquisitionGlobals.vi" "Acquiring?"() -> (w450:bool)
          }
          frame #1 {
            n321 = case shown="True" w462 {
              tunnel: w464 -> [_ w466]
              tunnel: w463 -> [_ w465]
              frame False {
              }
              frame True {
                n322 = Send Notification(notification=w465, notifier=w466) -> ()  [unwired: 1 in, 2 out]
              }
            }
          }
        }
      }
      event "Exposure Time": Value Change {
        n323 = event-data() -> ()  [unwired: 1 in, 6 out]
        n324 = flat-sequence {
          tunnel: w468 -> [w478]
          tunnel: [w470] -> w467
          frame #0 {
            n325 = property on="Exposure Time" class="Enum (strict)"() -> ("Strings []"=w477:string[])  [unwired: 2 in, 2 out]
            n326 = Decimal String To Number(string=w477) -> (number=w475:i32[])  [unwired: 2 in, 1 out]
            n327 = Index Array(array=w475, index="Exposure Time") -> (element=w474:i32)
            n328 = Divide(x=w474, y=1000.0) -> (x/y=w472:dbl)
            n329 = call <userlib>:"SetExposureTime.vi"("error in (no error)"=w478, "time"=w472) -> ("error out"=w471:errorcluster)  [unwired: 1 out]
            n330 = call "GetRealExposureTime.vi"("error in (no error)"=w471) -> ("error out"=w470:errorcluster, "Actual Exposure Time (ms)"=w469:dbl)  [unwired: 9 in]
            "Exposure Out" <- w469
            n331 = global write "LiveImage_Global.vi" "Exposure Time"(w469) -> ()
          }
        }
      }
      event "Piezo Position": Mouse Wheel {
        n332 = event-data() -> ("Delta"=w479:i32)  [unwired: 1 in, 9 out]
        n333 = flat-sequence {
          tunnel: w479 -> [w493]
          tunnel: [w486] -> w482
          tunnel: [w484] -> w480
          tunnel: w482 -> [w499]
          tunnel: w481 -> [w498]
          tunnel: w480 -> [w497]
          frame #0 {
            n334 = Sign(1:w493) -> (0:w491:i32)
            n335 = local read "Piezo Position"() -> (w496:dbl)
            n336 = global read "StateGlobals.vi" "Experiment State"() -> (w487:T3)
            n337 = Multiply(x=w491, y=0.1 ("x")) -> (x*y=w490:dbl)
            n338 = Add(x=w490, y=w496) -> (x+y=w489:dbl)
            "Piezo Position" <- w489
            n339 = Bundle By Name(cluster=w487, "Start or New Parameters?"=FALSE, "Begin Or End Acquisition"="ChangeDaq") -> (w486:T3)
            n340 = local write "Current Z Position (um)"(w489) -> ()
            n341 = Divide(x=w489, y=20.0) -> (x/y=w494:dbl)
            n342 = global write "StateGlobals.vi" "Experiment State"(w486) -> ()
            n343 = global write "NIDAQGlobals.vi" "Static Piezo Position"(w494) -> ()
            n344 = global read "AcquisitionGlobals.vi" "Acquiring?"() -> (w484:bool)
          }
          frame #1 {
            n345 = case shown="True" w497 {
              tunnel: w499 -> [_ w501]
              tunnel: w498 -> [_ w500]
              frame False {
              }
              frame True {
                n346 = Send Notification(notification=w501, notifier=w500) -> ()  [unwired: 1 in, 2 out]
              }
            }
          }
        }
      }
      event "Piezo Position": Value Change {
        n347 = event-data() -> ("NewVal"=w505:dbl)  [unwired: 1 in, 5 out]
        n348 = flat-sequence {
          tunnel: w505 -> [w511]
          tunnel: [w507] -> w504
          tunnel: [w506] -> w502
          tunnel: w504 -> [w516]
          tunnel: w503 -> [w515]
          tunnel: w502 -> [w514]
          frame #0 {
            n349 = global read "StateGlobals.vi" "Experiment State"() -> (w509:T3)
            n350 = Divide(x=w511, y=20.0) -> (x/y=w512:dbl)
            n351 = global write "NIDAQGlobals.vi" "Static Piezo Position"(w512) -> ()
            n352 = Bundle By Name(cluster=w509, "Start or New Parameters?"=FALSE, "Begin Or End Acquisition"="ChangeDaq") -> (w507:T3)
            n353 = global write "StateGlobals.vi" "Experiment State"(w507) -> ()
            n354 = global read "AcquisitionGlobals.vi" "Acquiring?"() -> (w506:bool)
          }
          frame #1 {
            n355 = case shown="True" w514 {
              tunnel: w516 -> [_ w518]
              tunnel: w515 -> [_ w517]
              frame False {
              }
              frame True {
                n356 = Send Notification(notification=w518, notifier=w517) -> ()  [unwired: 1 in, 2 out]
              }
            }
          }
        }
      }
    }
    "error out" <- w83
  }
  "Improper \nRange!" <- w2
